vi "Generate Code.vi"(8 "error in (no error)":errorcluster, 11 "RIO Target in":refnum<class "RIO Target.lvclass">) -> (0 "error out":errorcluster, 3 "RIO Target out":refnum<class "RIO Target.lvclass">)   [LabVIEW 2014, in "RIO Target.lvclass"]
uses:
  RIO Target.lvclass
  Scripting/Initialization Scripting/Initialization and IO Node Scripting.lvlib
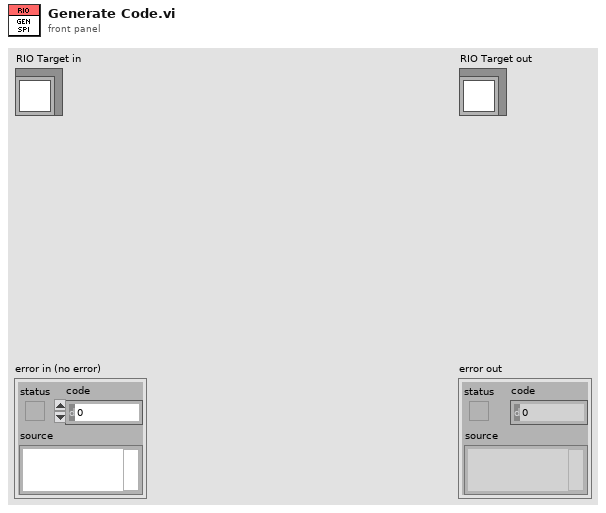
[diagram p1: front panel]
types:
  T1 = typedef "Input Paths.ctl" = cluster{"Golden Template (Source) - (make relative)":path, "Destination Generated Code (make relative)":path, "LabVIEW Project to Script":path, "VI to which to Add Engines and IO Nodes":path}
  T2 = typedef "Initialization and IO Node Scripting.lvlib/Bus Information.ctl" = cluster{"Devices":T3[], "Pin Information":T4, "Replacement VI for DLU":path, "Replacement VI for SPI Engine":path}
  T3 = typedef "Device Information.ctl" = cluster{"Number of Channels":i32, "Device Alias":string, "Device Icon Name":string[]}
  T4 = typedef "Pin Information.ctl" = cluster{"List of IO Names":string[], "List of Enable Lines":string[]}
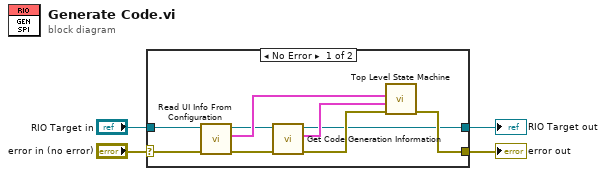
[diagram p0: block diagram]
diagram:
  n1 = case shown="No Error" "error in (no error)" {
    selector: "error in (no error)" -> [w12 w15]
    tunnel: [w13 w15] -> w3
    tunnel: [w5 w14] -> w1
    tunnel: "RIO Target in" -> [w11 w14]
    frame No Error {
      n2 = call "Read UI Info From Configuration.vi"("error in (no error)"=w12, "node in"=w11) -> ("error out"=w8:errorcluster, "Input Paths"=w10:T1, "node out"=w7:refnum<class "RIO Target.lvclass">)  [unwired: 6 in, 1 out]
      n3 = call "Get Code Generation Information.vi"("error in (no error)"=w8, "RIO Target in"=w7) -> ("error out"=w6:errorcluster, "Bus Information Array"=w9:T2[], "RIO Target out"=w5:refnum<class "RIO Target.lvclass">)  [unwired: 7 in]
      n4 = call "Top Level State Machine.vi"("error in"=w6, "Buses"=w9, "Input Paths"=w10) -> ("error out"=w13:errorcluster)  [unwired: 8 in]
    }
    frame Error {
    }
  }
  "error out" <- w3
  "RIO Target out" <- w1
